vi "Initialize.vi"(8 "error in (no error)":errorcluster, 11 "Stage_MadCityLab in":refnum<class "Stage_MadCityLab.lvclass">) -> (0 "error out":errorcluster, 3 "Stage_MadCityLab out":refnum<class "Stage_MadCityLab.lvclass">)   [LabVIEW 2020, in "Stage_MadCityLab.lvlib" / "Stage_MadCityLab.lvclass"]
uses:
  Stage_MadCityLab.lvclass
  Stage_MadCityLab.lvclass/Stage_MadCityLab.ctl
  Hardware Abstraction Layer/Component/Stage/Stage/Stage.lvclass
  Dependency/Madlib.dll
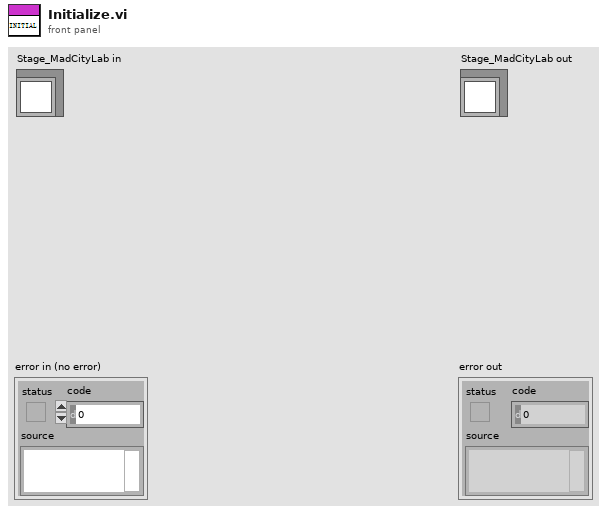
[diagram p1: front panel]
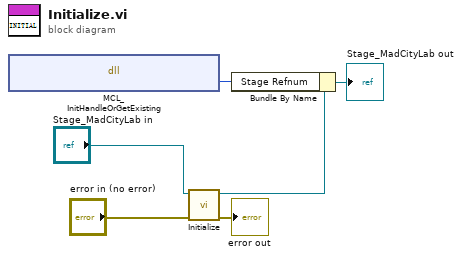
[diagram p0: block diagram]
diagram:
  n1 = dll-call lib="E:/Development/DevHardSoftware/MicroscopyFramework/Model/Hardware Layer/Real Hardware/Stage_MadCityLab/Stage_MadCityLab/Dependency/Madlib.dll" fn="MCL_InitHandleOrGetExisting"() -> ("return type"=w4:i32)  [unwired: 3 in, 2 out]
  n2 = call-parent "Initialize.vi"("error in (no error)"="error in (no error)", "Device in"="Stage_MadCityLab in") -> ("error out"=→"error out":errorcluster, "Device out"=w2:refnum<class "Stage_MadCityLab.lvclass">)  [unwired: 8 in]
  n3 = Bundle By Name(cluster=w2, "Stage Refnum"=w4) -> (→"Stage_MadCityLab out":refnum<class "Stage_MadCityLab.lvclass">)
